vi "State Entry.vi"(8 "error in (no error)":errorcluster, 11 "View Model":T1) -> (0 "error out":errorcluster, 3 "View Model":T1)   [LabVIEW 2017]
doc: "Initializes state information at beginning of transition"
uses:
  View Model/Controls/View Model.ctl
  Error Handler/Controls/Error Model.ctl
  Error Handler/Controls/Error EventData.ctl
  Error Handler/Controls/Error Type.ctl
  Controls/Elevator Model.ctl
  Controls/Elevator Overhead.ctl
  Controls/Elevator States.ctl
  Controls/Elevator Location.ctl
  Controls/Elevator Command Event.ctl
  Controls/Elevator Commands.ctl
  Configuration/Controls/Configuration Model.ctl
  Configuration/Controls/Configuration Data.ctl
  View Model/Controls/Shared Model.ctl
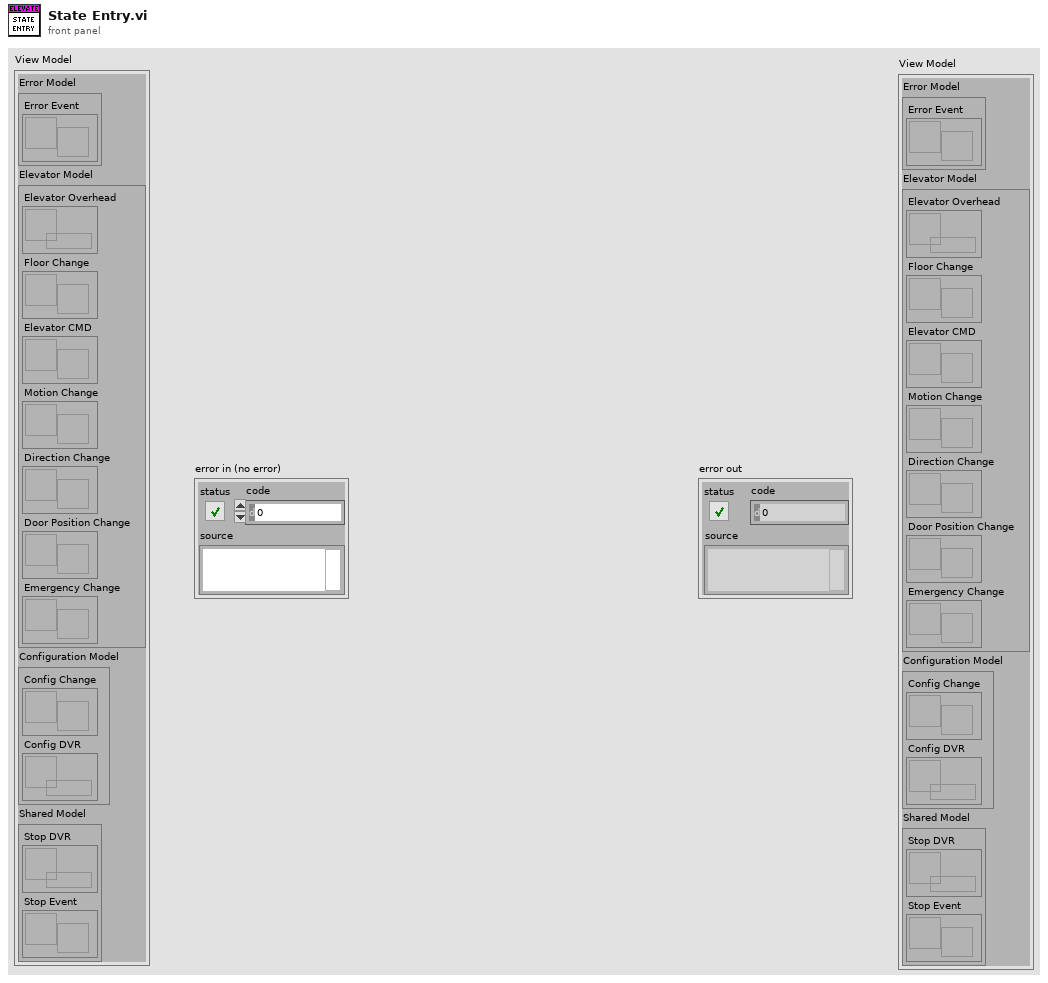
[diagram p1: front panel]
types:
  T1 = typedef "View Model.ctl" = cluster{"Error Model":T2, "Elevator Model":T3, "Configuration Model":T4, "Shared Model":T5}
  T2 = typedef "Error Model.ctl" = cluster{"Error Event":refnum<user-event>}
  T3 = typedef "Elevator Model.ctl" = cluster{"Elevator Overhead":refnum<data-value>, "Floor Change":refnum<user-event>, "Elevator CMD":refnum<user-event>, "Motion Change":refnum<user-event>, "Direction Change":refnum<user-event>, "Door Position Change":refnum<user-event>, "Emergency Change":refnum<user-event>}
  T4 = typedef "Configuration Model.ctl" = cluster{"Config Change":refnum<user-event>, "Config DVR":refnum<data-value>}
  T5 = typedef "Shared Model.ctl" = cluster{"Stop DVR":refnum<data-value>, "Stop Event":refnum<user-event>}
  T6 = typedef "Elevator States.ctl" = enum16{"Idle", "Init", "Open Doors", "Close Doors", "Start Move", "Move", "Finish Move", "Analysis", "Emergency"}
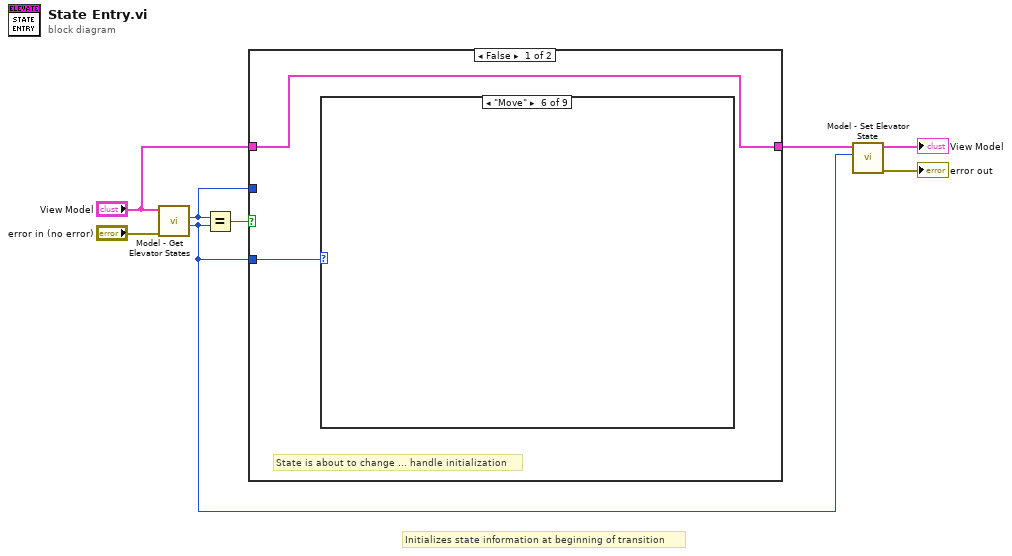
[diagram p0: block diagram]
diagram:
  # "Initializes state information at beginning of transition"
  n1 = call "Model - Get Elevator States.vi"("error in (no error)"="error in (no error)", "View Model"="View Model") -> ("Next Elevator State"=w4:T6, "Elevator State"=w6:T6)  [unwired: 6 in, 2 out]
  n2 = Equal?(x=w6, y=w4) -> (x = y?=w8:bool)
  n3 = case shown="False" w8 {
    tunnel: "View Model" -> [w9 w11]
    tunnel: w4 -> [w10 _]
    tunnel: w6 -> [_ _]
    tunnel: [w9 w11] -> w5
    frame False {
      # "State is about to change ... handle initialization"
      n4 = case shown="\"Move\"" w10 {
        frame "Idle", Default {
        }
        frame "Init" {
        }
        frame "Open Doors" {
          # "[Covers: OC3A]"
          # "[Covers: OC3]"
          # "Start open door timer"
        }
        frame "Close Doors" {
        }
        frame "Start Move" {
          # "[Covers: OC6]"
          # "Fire a motion event"
          # "[Covers: CT1]"
          # "[Covers: SS4]"
          # "Initialize travel timer in view model"
        }
        frame "Move" {
        }
        frame "Finish Move" {
        }
        frame "Analysis" {
        }
        frame "Emergency" {
        }
      }
    }
    frame True {
    }
  }
  n5 = call "Model - Set Elevator State.vi"("Elevator State"=w4, "View Model"=w5) -> ("error out"=→"error out":errorcluster, "View Model"=→"View Model":T1)  [unwired: 8 in]
